vi "Log Data Scan Mode.vi"() -> ()   [LabVIEW 2023]
uses:
  <vilib>/Platform/TimedLoop/XDataNode/timing_clust.ctl
  <vilib>/Platform/TimedLoop/XDataNode/nitl_modes.ctl
  <vilib>/Platform/TimedLoop/XDataNode/wakeup.ctl
  <vilib>/platform/TimedLoop/XDataNode/XDataNode.xnode
  <vilib>/Platform/TimedLoop/XDataNode/XDNodeRunTimeDep.lvlib
panel:
  in  "file path":path
  in  "Stop":bool
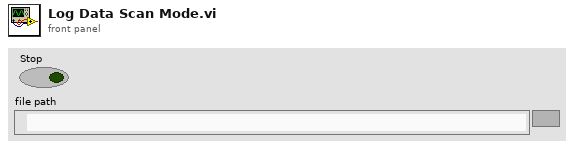
[diagram p1: front panel]
types:
  T1 = enum16{"open", "open or create", "create or replace", "create", "open (read-only)"}
  T2 = typedef "XDNodeRunTimeDep.lvlib/timing_clust.ctl" = cluster{"Expected End [f-1]":u64, "Actual End [f-1]":u64, "Finished Late? [f-1]":bool, "Expected End [i-1]":u64, "Actual End [i-1]":u64, "Finished Late? [i-1]":bool, "Expected Start [i]":u64, "Actual Start [i]":u64, "Expected Start [f]":u64, "Actual Start [f]":u64, "Source Name":string, "Structure Name":string, "Period":i64, "Deadline":i64, "Offset":i64, "Start":i64, "Priority":i32, "Timeout":i32, "Mode":T3, "Wakeup Reason":T4, "Error":errorcluster, "Source Type":string, "Secondary Source Type":string, "Global End Time":u64, "Global Start Time":u64, "Frame Duration":u64, "Iteration Duration":u64, "Assigned CPU":i32, "I/O Scan Engine Mode":u32}
  T3 = typedef "XDNodeRunTimeDep.lvlib/nitl_modes.ctl" = enum32{"No Change", "Process missed periods, maintain original phase", "Discard missed periods, maintain original phase", "Process missed periods, ignore original phase", "Discard missed periods, ignore original phase"}
  T4 = typedef "XDNodeRunTimeDep.lvlib/wakeup.ctl" = enum32{"Normal", "Aborted", "Asynchronous wakeup", "Timing source error", "Timed loop error", "Timeout"}
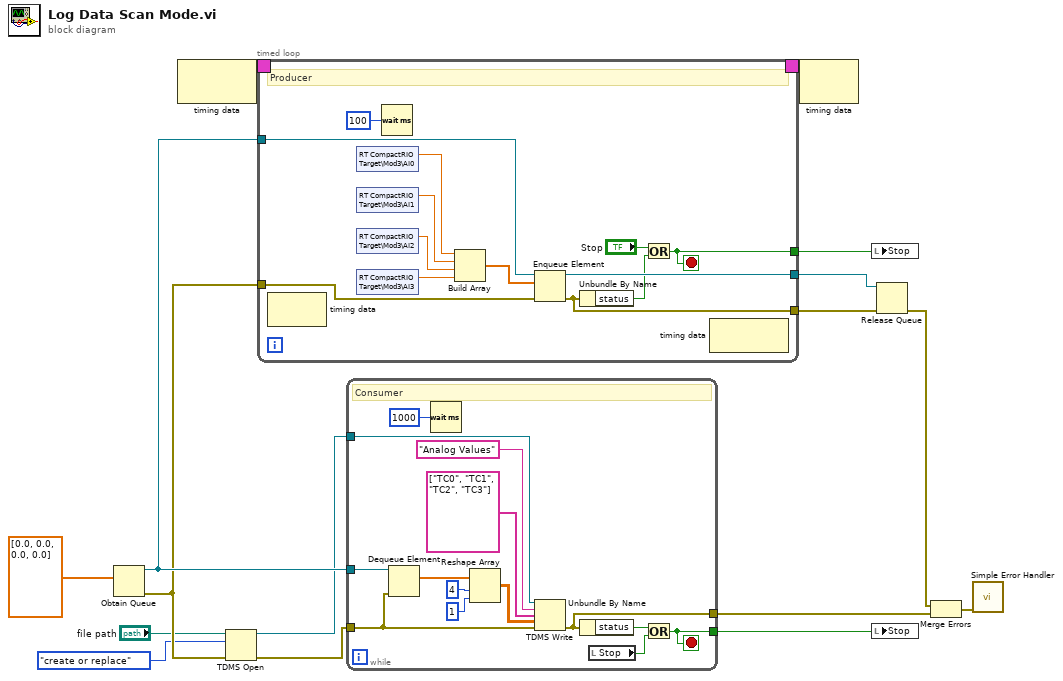
[diagram p0: block diagram]
diagram:
  n1 = Obtain Queue(element data type=dbl[] [0.0, 0.0, 0.0, 0.0] ("appended array 3")) -> (queue out=w14:refnum<queue>, error out=w12:errorcluster)  [unwired: 4 in, 1 out]
  n2 = node-c288() -> (w11:T2)  [unwired: 1 in]
  n3 = TDMS Open(8:w12, 10:T1."create or replace" ("operation (0:open)"), 11:"file path") -> (0:w13:errorcluster, 3:w9:refnum<k34>)  [unwired: 4 in]
  n4 = timed-loop {
    tunnel: w12 -> [w29]
    tunnel: w14 -> [w28]
    tunnel: [w26] -> w16
    tunnel: [w27] -> w15
    timing: w11 -> [_]
    timing-out: [_] -> w10
    tunnel: [w22] -> w8
    stop <- w22 stop-if-true
    # "Producer"
    n5 = node-c288() -> ()  [unwired: 1 in, 1 out]
    n6 = shared-variable "RT CompactRIO Target\\Mod3\\AI0"() -> (w18:dbl)  [unwired: 1 in, 1 out]
    n7 = shared-variable "RT CompactRIO Target\\Mod3\\AI1"() -> (w19:dbl)  [unwired: 1 in, 1 out]
    n8 = shared-variable "RT CompactRIO Target\\Mod3\\AI2"() -> (w20:dbl)  [unwired: 1 in, 1 out]
    n9 = shared-variable "RT CompactRIO Target\\Mod3\\AI3"() -> (w21:dbl)  [unwired: 1 in, 1 out]
    n10 = Wait (ms)(milliseconds to wait=u32 100) -> ()  [unwired: 1 out]
    n11 = Build Array(w18, w19, w20, w21) -> (w17:dbl[])
    n12 = Enqueue Element(queue=w28, element=w17, error in (no error)=w29) -> (queue out=w27:refnum<queue>, error out=w26:errorcluster)  [unwired: 1 in, 1 out]
    n13 = Unbundle By Name(w26) -> ("status"=w25:bool)
    n14 = Or(x="Stop", y=w25) -> (x .or. y?=w22:bool)
    n15 = node-c288() -> ()  [unwired: 1 in, 1 out]
  }
  n16 = while {
    tunnel: w14 -> [w45]
    tunnel: w13 -> [w44]
    tunnel: w9 -> [w43]
    tunnel: [w40] -> w7
    tunnel: [w39] -> w6
    stop <- w40 stop-if-true
    # "Consumer"
    n17 = Dequeue Element(queue=w45, error in (no error)=w44) -> (element=w38:dbl[])  [unwired: 1 in, 3 out]
    n18 = Wait (ms)(milliseconds to wait=u32 1000) -> ()  [unwired: 1 out]
    n19 = Reshape Array(w38, 4 ("dimension size"), 1 ("dimension size")) -> (w32:dbl[][])
    n20 = TDMS Write(0:w43, 5:"Analog Values" ("group name in (Untitled)"), 7:string[] ["TC0", "TC1", "TC2", "TC3"] ("channel name(s) in (Untitled)"), 9:w32, 11:w44) -> (15:w39:errorcluster)  [unwired: 1 in, 3 out]
    n21 = Unbundle By Name(w39) -> ("status"=w42:bool)
    n22 = local read "Stop"() -> (w41:bool)
    n23 = Or(x=w42, y=w41) -> (x .or. y?=w40:bool)
  }
  n24 = node-c288(w10) -> ()  [unwired: 1 out]
  n25 = local write "Stop"(w8) -> ()
  n26 = local write "Stop"(w7) -> ()
  n27 = Release Queue(queue=w15, error in (no error)=w16) -> (error out=w5:errorcluster)  [unwired: 1 in, 2 out]
  n28 = Merge Errors(w5, w6) -> (w4:errorcluster)
  n29 = call <vilib>:"Simple Error Handler.vi"("error in (no error)"=w4) -> ()  [unwired: 4 in, 5 out]
